vi "LVDimInterface.test ping pong server.vi"() -> ()   [LabVIEW 2015, in "LVDimInterface.lvlib"]
doc: "This VI implements a DIM server, that publishes a loop counter as a DIM service"
uses:
  LVDimInterface.lvlib
  LVDimInterface.dis_add_command_queue.vi
panel:
  out "error out":errorcluster
  in  "commandName":string="testCommand"
  out "throughput [kBytes/s]":dbl
  out "updateRate [Hz]":dbl
  in  "nOfBuffers":i32=100
  in  "bufferSize":i32=10
  out "bufferCounter":i32
  in  "serverName":string="simpleServer"
  in  "serviceName":string="testBuffer"
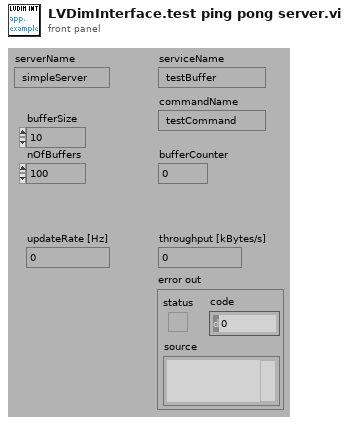
[diagram p1: front panel]
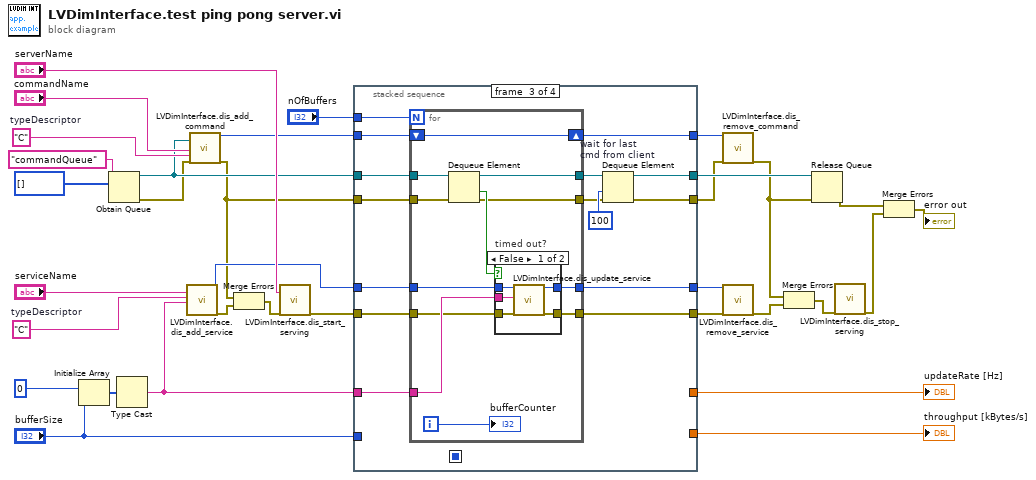
[diagram p0: block diagram]
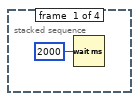
[diagram p2: hidden frame]
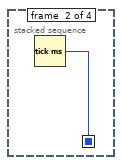
[diagram p3: hidden frame]
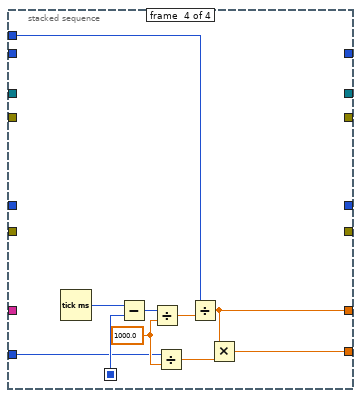
[diagram p5: hidden frame]
diagram:
  w16 = "C"  # typeDescriptor
  w28 = "C"  # typeDescriptor
  n1 = Initialize Array(i8 0 ("defaultData"), "bufferSize") -> (w25:i8[])
  n2 = Obtain Queue(name (unnamed)="commandQueue", element data type=i8[] []) -> (queue out=w14:refnum<queue>, error out=w8:errorcluster)  [unwired: 3 in, 1 out]
  n3 = Type Cast(x=w25) -> (*(type *) &x=w20:string)  [unwired: 1 in]
  n4 = call "LVDimInterface.dis_add_service.vi"("serviceName"="serviceName", "typeDescriptor"=w28, "data"=w20) -> ("my_serviceID"=w27:i32, "error out"=w4:errorcluster)  [unwired: 15 in]
  n5 = call-poly "LVDimInterface.dis_add_command.vi"("queueRef"=w14, "commandName"="commandName", "typeDescriptor"=w16, "error in (no error)"=w8) -> ("commandID"=w15:i32, "error out"=w5:errorcluster)  [unwired: 14 in]
  n6 = Merge Errors(w5, w4) -> (w6:errorcluster)
  n7 = call "LVDimInterface.dis_start_serving.vi"("serverName"="serverName", "error in (no error)"=w6) -> ("error out"=w31:errorcluster)  [unwired: 16 in, 1 out]
  n8 = stacked-sequence {
    seq-local: [_ w35 _ _] -> [_ _ _ w78]
    tunnel: [_ _ w50 _] -> w33
    tunnel: w31 -> [_ _ w49 _]
    tunnel: [_ _ w48 _] -> w30
    tunnel: w27 -> [_ _ w47 _]
    tunnel: w20 -> [_ _ w46 _]
    tunnel: "nOfBuffers" -> [_ _ w45 w76]
    tunnel: "bufferSize" -> [_ _ _ w73]
    tunnel: [_ _ _ w71] -> w22
    tunnel: [_ _ _ w70] -> w21
    tunnel: w15 -> [_ _ w43 _]
    tunnel: w14 -> [_ _ w44 _]
    tunnel: [_ _ w41 _] -> w10
    tunnel: [_ _ w39 _] -> w13
    tunnel: w5 -> [_ _ w38 _]
    tunnel: [_ _ w36 _] -> w7
    frame #0 {
      n9 = Wait (ms)(milliseconds to wait=u32 2000) -> ()  [unwired: 1 out]
    }
    frame #1 {
      n10 = Tick Count (ms)() -> (millisecond timer value=w35:u32)
    }
    frame #2 {
      n11 = for {
        N: w45 -> [_]
        tunnel: [w62] -> w50
        tunnel: w49 -> [w57]
        tunnel: [w60] -> w48
        tunnel: w47 -> [w58]
        tunnel: w46 -> [w59]
        tunnel: w44 -> [w56]
        tunnel: [w54] -> w42
        shift-right: [w53] -> w39
        shift-left: w43 -> [w53]
        tunnel: w38 -> [w52]
        tunnel: [w51] -> w37
        i -> [w61]
        n12 = Dequeue Element(queue=w56, error in (no error)=w52) -> (queue out=w54:refnum<queue>, timed out?=w55:bool, error out=w51:errorcluster)  [unwired: 1 in, 1 out]
        n13 = case "timed out?" shown="False" w55 {
          tunnel: [w67 w69] -> w62
          tunnel: [w66 w68] -> w60
          tunnel: w59 -> [w65 _]
          tunnel: w58 -> [w64 w69]
          tunnel: w57 -> [w63 w68]
          frame False {
            n14 = call "LVDimInterface.dis_update_service.vi"("my_serviceID"=w64, "data"=w65, "error in (no error)"=w63) -> ("my_serviceID out"=w67:i32, "error out"=w66:errorcluster)  [unwired: 14 in, 1 out]
          }
          frame True {
          }
        }
        "bufferCounter" <- w61
      }
      n15 = Dequeue Element "wait for last\ncmd from client"(queue=w42, timeout in ms (-1)=100, error in (no error)=w37) -> (queue out=w41:refnum<queue>, error out=w36:errorcluster)  [unwired: 2 out]
    }
    frame #3 {
      w74 = 1000.0 ("y")
      n16 = Tick Count (ms)() -> (millisecond timer value=w79:u32)
      n17 = Subtract(x=w79, y=w78) -> (x-y=w77:u32)
      n18 = Divide(x=w77, y=w74) -> (x/y=w75:dbl)
      n19 = Divide(x=w73, y=w74) -> (x/y=w72:dbl)
      n20 = Divide(x=w76, y=w75) -> (x/y=w71:dbl)
      n21 = Multiply(x=w71, y=w72) -> (x*y=w70:dbl)
    }
  }
  "updateRate [Hz]" <- w22
  "throughput [kBytes/s]" <- w21
  n22 = call "LVDimInterface.dis_remove_command.vi"("commandID"=w13, "error in (no error)"=w7) -> ("error out"=w9:errorcluster)  [unwired: 17 in]
  n23 = call "LVDimInterface.dis_remove_service.vi"("my_serviceID"=w33, "error in (no error)"=w30) -> ("error out"=w11:errorcluster)  [unwired: 17 in]
  n24 = Merge Errors(w9, w11) -> (w12:errorcluster)
  n25 = Release Queue(queue=w10, error in (no error)=w9) -> (error out=w3:errorcluster)  [unwired: 1 in, 2 out]
  n26 = call "LVDimInterface.dis_stop_serving.vi"("error in (no error)"=w12) -> ("error out"=w2:errorcluster)  [unwired: 18 in]
  n27 = Merge Errors(w3, w2) -> (→"error out":errorcluster)
